vi "PID File Read.vi"   [LabVIEW 2013]
uses:
  Team Code/Robot Global Data.vi
types:
  T1 = cluster{"Output Value":dbl, "Output Value":dbl, "Output Value":dbl}
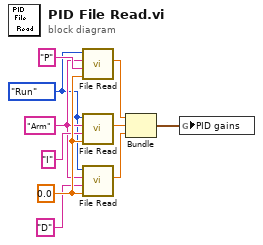
[diagram p0: block diagram]
diagram:
  w6 = 0.0 ("Default Value")
  w2 = "Arm" ("section")
  w1 = enum16{"Init", "Run", "End"}."Run" ("Mode")
  n1 = call "File Read.vi"("Default Value"=w6, "key"="P", "section"=w2, "Mode"=w1) -> ("Output Value"=w7:dbl)  [unwired: 7 out]
  n2 = call "File Read.vi"("Default Value"=w6, "key"="I", "section"=w2, "Mode"=w1) -> ("Output Value"=w8:dbl)  [unwired: 7 out]
  n3 = call "File Read.vi"("Default Value"=w6, "key"="D", "section"=w2, "Mode"=w1) -> ("Output Value"=w9:dbl)  [unwired: 7 out]
  n4 = Bundle("Output Value"=w7, "Output Value"=w8, "Output Value"=w9) -> (w10:T1)  [unwired: 1 out]
  n5 = global write "Robot Global Data.vi" "PID gains"(w10) -> ()
